vi "Init.vi"(8 "error in (no error)":errorcluster, 11 "Coca Actors in":refnum<class "Coca Actors.lvclass">) -> (0 "error out":errorcluster, 3 "Coca Actors out":refnum<class "Coca Actors.lvclass">)   [LabVIEW 2020, in "Coca Actors.lvlib" / "Coca Actors.lvclass"]
uses:
  Coca Actors.lvclass
  Coca Actors.lvclass/Coca Actors.ctl
  <vilib>/Utility/config.llb/Read Key (Double).vi
  <vilib>/Utility/config.llb/Read Key (String).vi
  <vilib>/Utility/config.llb/NI_LVConfig.lvlib
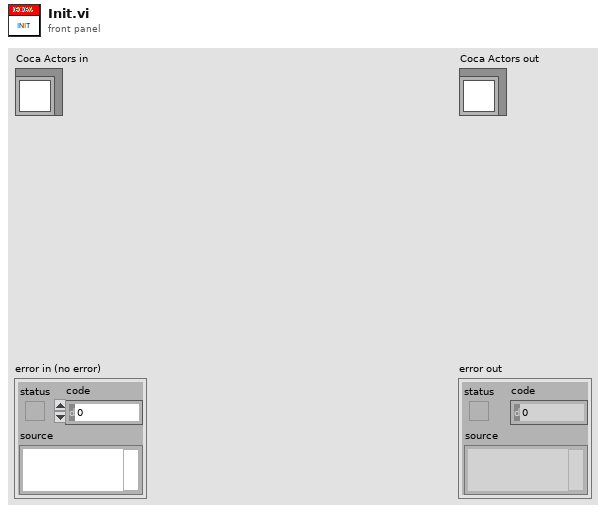
[diagram p1: front panel]
types:
  T1 = typedef "NI_LVConfig.lvlib/Config Data RefNum.ctl" = refnum<k1>
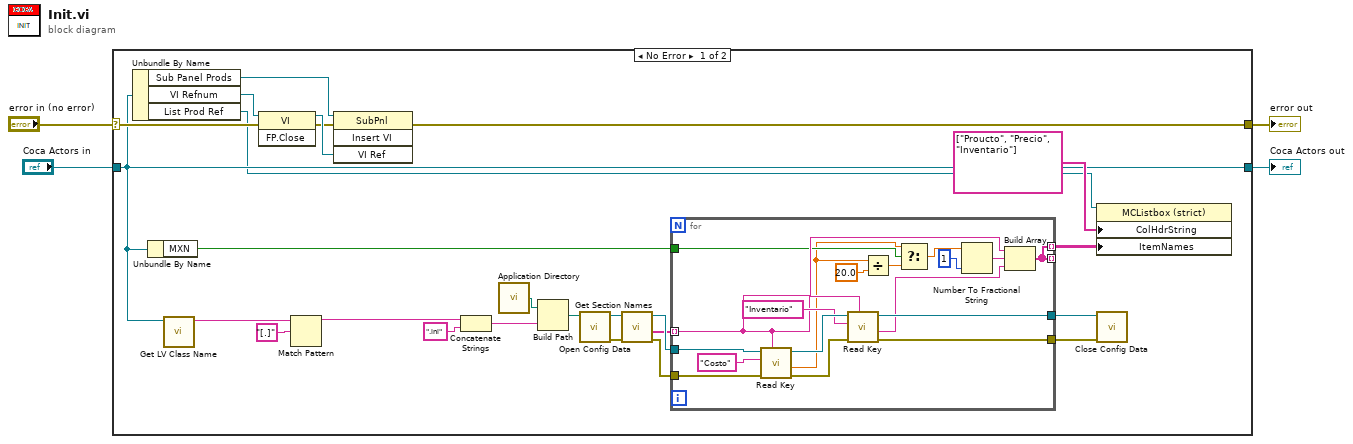
[diagram p0: block diagram]
diagram:
  n1 = case shown="No Error" "error in (no error)" {
    selector: "error in (no error)" -> [w25 w49]
    tunnel: [w24 w49] -> w3
    tunnel: [w12 w48] -> w1
    tunnel: "Coca Actors in" -> [w12 w48]
    frame No Error {
      n2 = Unbundle By Name(w12) -> ("Sub Panel Prods"=w28:refnum<vi>, "VI Refnum"=w29:refnum<vi>, "List Prod Ref"=w6:refnum<vi>)
      n3 = Unbundle By Name(w12) -> ("MXN"=w11:bool)
      n4 = call <vilib>:"Get LV Class Name.vi"("object"=w12) -> ("class name"=w15:string)  [unwired: 9 in, 1 out]
      n5 = invoke class="VI" method="FP.Close"(reference=w29, error in=w25) -> (reference out=w27:refnum<vi>, error out=w26:errorcluster)  [unwired: 1 in, 1 out]
      n6 = Match Pattern(string=w15, regular expression="[.]") -> (before substring=w14:string)  [unwired: 1 in, 3 out]
      n7 = invoke class="SubPnl" method="Insert VI"(reference=w28, error in=w26, "VI Ref"=w27) -> (error out=w24:errorcluster)  [unwired: 1 in, 3 out]
      n8 = Concatenate Strings(w14, ".ini" ("string")) -> (w21:string)
      n9 = call <vilib>:"Application Directory.vi"() -> ("Application Directory"=w22:path)
      n10 = Build Path(base path=w22, name or relative path=w21) -> (appended path=w19:path)
      n11 = call <vilib>:"Open Config Data.vi"("configuration file path"=w19) -> ("error out"=w18:errorcluster, "refnum"=w9:T1)  [unwired: 8 in, 1 out]
      n12 = call <vilib>:"Get Section Names.vi"("error in (no error)"=w18, "refnum"=w9) -> ("error out"=w10:errorcluster, "section names"=w7:string[], "refnum out"=w8:T1)  [unwired: 7 in]
      n13 = for {
        tunnel: w8 -> [w47]
        tunnel: w10 -> [w46]
        tunnel: [w42] -> w17
        tunnel: [w43] -> w16
        tunnel: w11 -> [w34]
        tunnel: w7 -> [w39] mode=indexing
        tunnel: [w37] -> _ mode=indexing
        tunnel: [w37] -> w5 mode=indexing
        n14 = call-poly <vilib>:"Read Key.vi"("section"=w39, "error in (no error)"=w46, "key"="Costo", "refnum"=w47) -> ("error out"=w44:errorcluster, "value"=w32:dbl, "refnum out"=w45:T1)  [unwired: 4 in, 1 out]
        n15 = call-poly <vilib>:"Read Key.vi"("section"=w39, "error in (no error)"=w44, "key"="Inventario", "refnum"=w45) -> ("error out"=w42:errorcluster, "value"=w38:string, "refnum out"=w43:T1)  [unwired: 4 in, 1 out]
        n16 = Divide(x=w32, y=20.0) -> (x/y=w30:dbl)
        n17 = Select(t=w32, s=w34, f=w30) -> (s? t:f=w33:dbl)
        n18 = Number To Fractional String(number=w33, precision (6)=i16 1) -> (F-format string=w35:string)  [unwired: 2 in]
        n19 = Build Array(w39, w35, w38) -> (w37:string[])
      }
      n20 = property class="MCListbox (strict)"(reference=w6, "ColHdrString"=string[] ["Proucto", "Precio", "Inventario"] ("Column Header Strings[]"), "ItemNames"=w5) -> ()  [unwired: 1 in, 2 out]
      n21 = call <vilib>:"Close Config Data.vi"("error in (no error)"=w17, "refnum"=w16) -> ()  [unwired: 8 in, 2 out]
    }
    frame Error {
    }
  }
  "error out" <- w3
  "Coca Actors out" <- w1
